vi "XML to Slope Calibration Inputs.vi"(0 "XML Data":string) -> ()   [LabVIEW 2013]
uses:
  Types/Slope Calibration Inputs.ctl
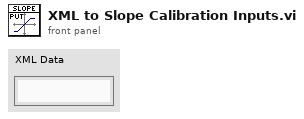
[diagram p1: front panel]
types:
  T1 = typedef "Slope Calibration Inputs.ctl" = cluster{"Number of Samples":dbl, "Ramp Rate":dbl, "Z Scan Size":dbl, "Version":string}
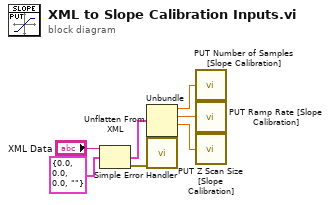
[diagram p0: block diagram]
diagram:
  n1 = Unflatten From XML(xml string="XML Data", type=T1 {"Number of Samples"=0.0, "Ramp Rate"=0.0, "Z Scan Size"=0.0, "Version"=""} ("Slope Calibration Inputs")) -> (value=w7:T1, error out=w4:errorcluster)  [unwired: 1 in]
  n2 = Unbundle(w7) -> ("Number of Samples"=w2:dbl, "Ramp Rate"=w3:dbl, "Z Scan Size"=w1:dbl)  [unwired: 1 out]
  n3 = call <vilib>:"Simple Error Handler.vi"("error in (no error)"=w4) -> ()  [unwired: 4 in, 5 out]
  n4 = call "PUT Number of Samples [Slope Calibration].vi"("Number of Samples"=w2) -> ()
  n5 = call "PUT Ramp Rate [Slope Calibration].vi"("Ramp Rate"=w3) -> ()
  n6 = call "PUT Z Scan Size [Slope Calibration].vi"("Z Scan Size"=w1) -> ()
